vi "Get Object Information.vi"(8 "error in (no error)":errorcluster, 11 "Object DAO in":refnum<class "Object DAO.lvclass">) -> (0 "error out":errorcluster, 2 "Object Information":T1, 3 "Object DAO out":refnum<class "Object DAO.lvclass">)   [LabVIEW 2020, in "Object DAO.lvclass"]
uses:
  Object DAO.lvclass
  Type Def/Object Information.ctl
  Object DAO.lvclass/Object DAO.ctl
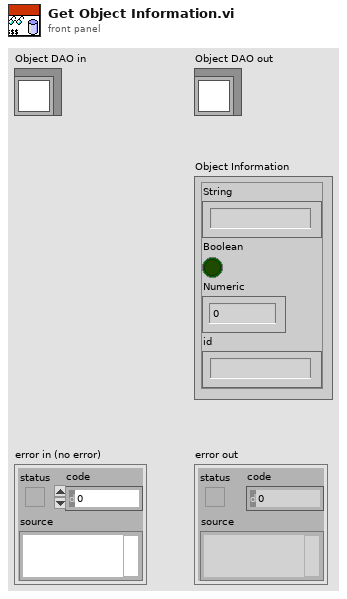
[diagram p1: front panel]
types:
  T1 = typedef "Object DAO.lvclass/Object Information.ctl" = cluster{"String":string, "Boolean":bool, "Numeric":dbl, "id":string}
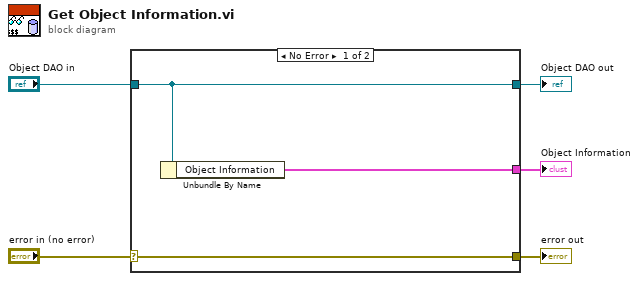
[diagram p0: block diagram]
diagram:
  n1 = case shown="No Error" "error in (no error)" {
    selector: "error in (no error)" -> [w8 w9]
    tunnel: [w8 w9] -> w4
    tunnel: [w7 w10] -> w2
    tunnel: "Object DAO in" -> [w7 w10]
    tunnel: [w6 _] -> w1
    frame No Error {
      n2 = Unbundle By Name(w7) -> ("Object Information"=w6:T1)
    }
    frame Error {
    }
  }
  "error out" <- w4
  "Object DAO out" <- w2
  "Object Information" <- w1
